vi "Telescope Init.vi"(8 "error in (no error)":errorcluster, 9 "Settings":variant, 10 "Name":string, 11 "PRIME Telescope in":refnum<class "PRIME Telescope.lvclass">) -> (0 "error out":errorcluster, 1 "Connect Message":string, 2 "Channel List":refnum<class "HK Item.lvclass">[](array[class]), 3 "PRIME Telescope out":refnum<class "PRIME Telescope.lvclass">)   [LabVIEW 2021, in "PRIME Telescope.lvclass"]
uses:
  PRIME Telescope.lvclass
  hk-channel-class/HK Item/HK Item.lvclass
  PRIME Telescope.lvclass/PRIME Telescope.ctl
  Telescope.lvclass
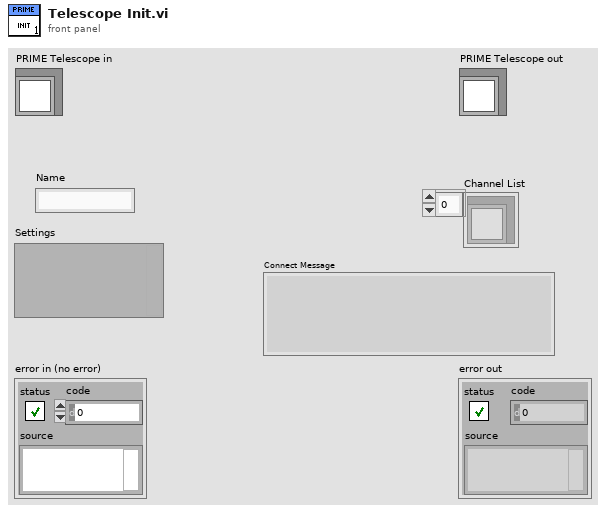
[diagram p1: front panel]
types:
  T1 = typedef "PRIME Telescope cluster Settings.ctl" = cluster{"IP Address":string, "port":u16}
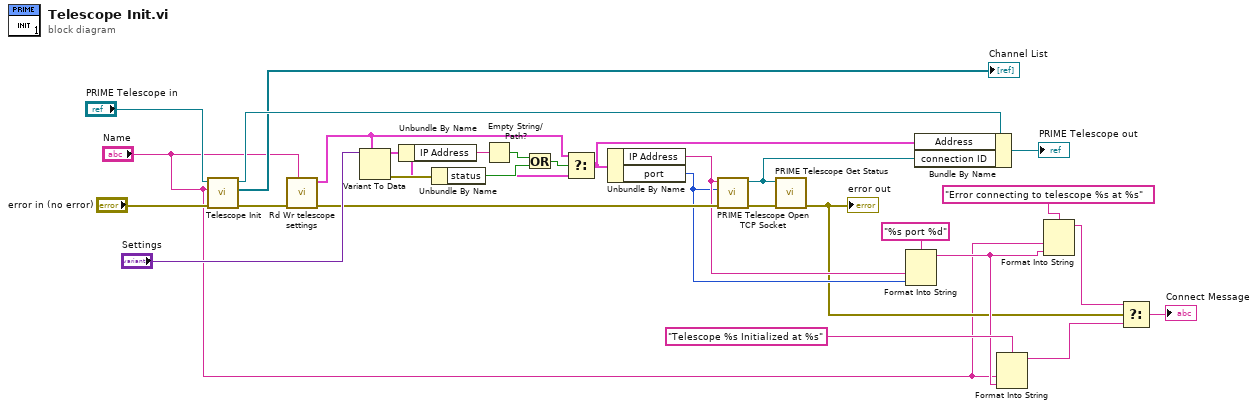
[diagram p0: block diagram]
diagram:
  n1 = call-parent "Telescope Init.vi"("error in (no error)"="error in (no error)", "Name"="Name", "Telescope in"="PRIME Telescope in") -> ("error out"=w16:errorcluster, "Channel List"=→"Channel List":refnum<class "HK Item.lvclass">[], "Telescope out"=w27:refnum<class "PRIME Telescope.lvclass">)  [unwired: 5 in, 1 out]
  n2 = call "Rd Wr telescope settings.vi"("Telescope Name"="Name", "error in (no error)"=w16) -> ("error out"=w15:errorcluster, "Telescope Settings"=w14:T1)  [unwired: 8 in]
  n3 = Variant To Data(type=w14, Variant="Settings") -> (data=w18:T1, error out=w21:errorcluster)  [unwired: 1 in]
  n4 = Unbundle By Name(w18) -> ("IP Address"=w24:string)
  n5 = Unbundle By Name(w21) -> ("status"=w20:bool)
  n6 = Empty String/Path?(string/path=w24) -> (empty?=w22:bool)
  n7 = Or(x=w22, y=w20) -> (x .or. y?=w23:bool)
  n8 = Select(t=w14, s=w23, f=w18) -> (s? t:f=w19:T1)
  n9 = Unbundle By Name(w19) -> ("IP Address"=w12:string, "port"=w11:u16)
  n10 = call "PRIME Telescope Open TCP Socket.vi"("error in (no error)"=w15, "port"=w11, "IP Address"=w12) -> ("error out"=w4:errorcluster, "connection ID"=w3:refnum<k5>)  [unwired: 7 in]
  n11 = call "PRIME Telescope Get Status.vi"("error in (no error)"=w4, "connection ID"=w3) -> ("error out"=w2:errorcluster)  [unwired: 5 in, 4 out]
  "error out" <- w2
  n12 = Format Into String(format string="%s port %d", w12, w11) -> (resulting string=w6:string)  [unwired: 2 in, 1 out]
  n13 = Bundle By Name(cluster=w27, "Address"=w19, "connection ID"=w3) -> (→"PRIME Telescope out":refnum<class "PRIME Telescope.lvclass">)
  n14 = Format Into String(format string="Telescope %s Initialized at %s", "Name", w6) -> (resulting string=w8:string)  [unwired: 2 in, 1 out]
  n15 = Format Into String(format string="Error connecting to telescope %s at %s", "Name", w6) -> (resulting string=w5:string)  [unwired: 2 in, 1 out]
  n16 = Select(t=w5, s=w2, f=w8) -> (s? t:f=→"Connect Message":string)
